vi "Create.vi"(8 "error in (no error)":errorcluster, 10 "Historian MsgQ":refnum<class "MessageQ.lvclass">) -> (0 "error out":errorcluster, 3 "History Data Controller out":refnum<class "History Data Controller.lvclass">)   [LabVIEW 2020, in "VolatusHistorian.lvlib" / "History Data Controller.lvclass"]
uses:
  History Data Controller.lvclass
  History Data Controller.lvclass/History Data Controller.ctl
  Volatus/MessageQ/MessageQ.lvclass
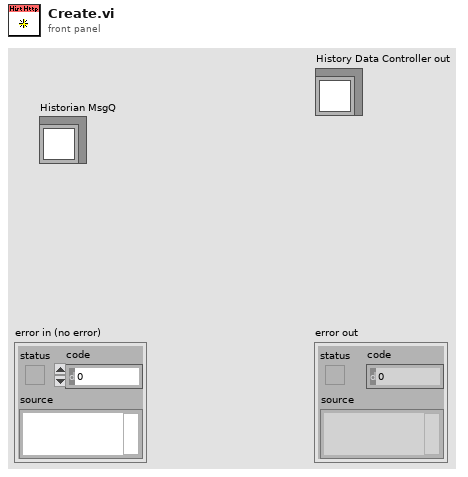
[diagram p1: front panel]
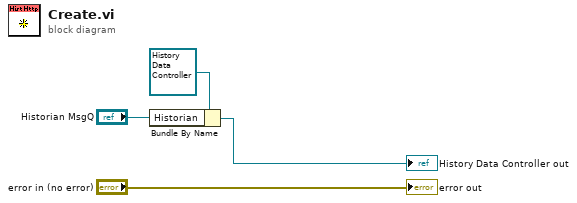
[diagram p0: block diagram]
diagram:
  n1 = Bundle By Name(cluster=refnum<class "History Data Controller.lvclass"> refnum ("History Data Controller in"), "Historian"="Historian MsgQ") -> (→"History Data Controller out":refnum<class "History Data Controller.lvclass">)
  "error out" <- "error in (no error)"
